vi "INIT.vi"(8 "error in (no error)":errorcluster, 11 "Mensajes in":refnum<class "Mensajes.lvclass">) -> (0 "error out":errorcluster, 3 "Mensajes out":refnum<class "Mensajes.lvclass">)   [LabVIEW 2019, in "Mensajes.lvlib" / "Mensajes.lvclass"]
uses:
  Mensajes.lvclass
  Mensajes.lvclass/Mensajes.ctl
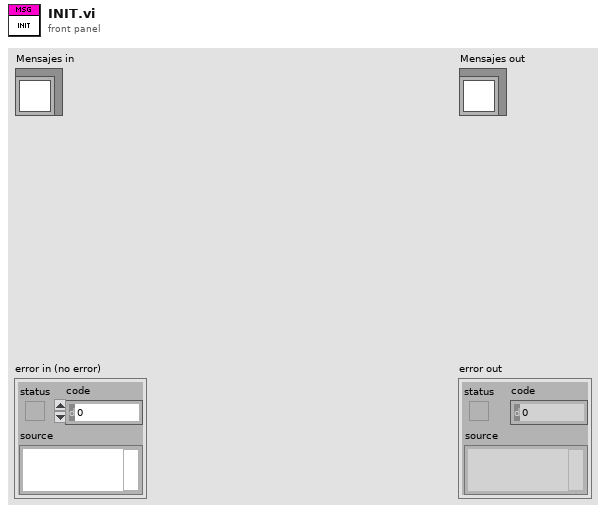
[diagram p1: front panel]
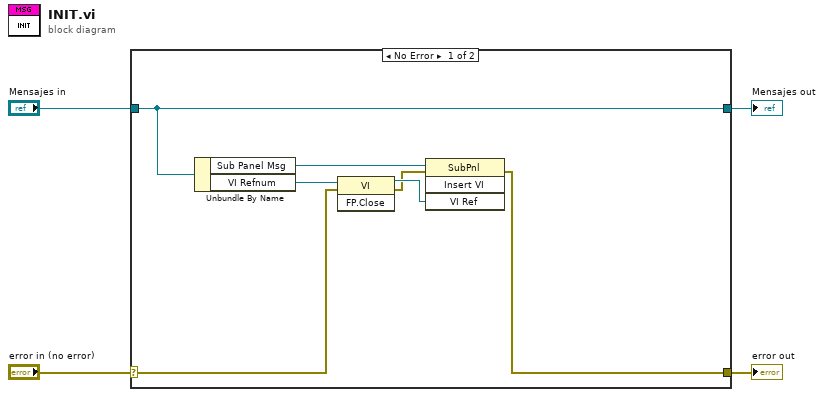
[diagram p0: block diagram]
diagram:
  n1 = case shown="No Error" "error in (no error)" {
    selector: "error in (no error)" -> [w7 w13]
    tunnel: [w6 w13] -> w3
    tunnel: [w8 w12] -> w1
    tunnel: "Mensajes in" -> [w8 w12]
    frame No Error {
      n2 = Unbundle By Name(w8) -> ("Sub Panel Msg"=w5:refnum<vi>, "VI Refnum"=w11:refnum<vi>)
      n3 = invoke class="VI" method="FP.Close"(reference=w11, error in=w7) -> (reference out=w10:refnum<vi>, error out=w9:errorcluster)  [unwired: 1 in, 1 out]
      n4 = invoke class="SubPnl" method="Insert VI"(reference=w5, error in=w9, "VI Ref"=w10) -> (error out=w6:errorcluster)  [unwired: 1 in, 3 out]
    }
    frame Error {
    }
  }
  "error out" <- w3
  "Mensajes out" <- w1
